vi "Create Controller Names.vi"(0 "Controller name":string, 11 "error in (no error)":errorcluster) -> (4 "Controller Names":string[](array[string]), 15 "error out":errorcluster)   [LabVIEW 2020]
doc: "Create a controller name array from given controller name.\n\nC-887: \nadd additional names for this controller."
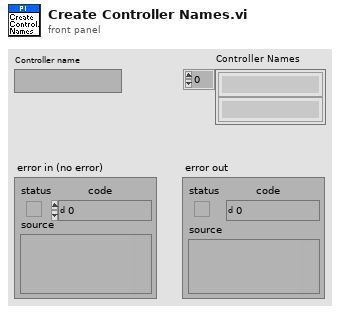
[diagram p1: front panel]
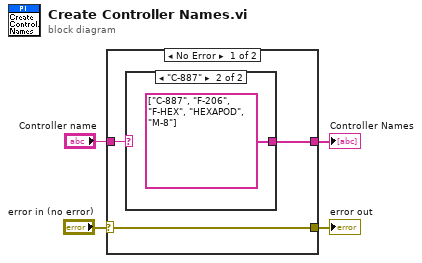
[diagram p0: block diagram]
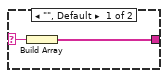
[diagram p2: hidden frame]
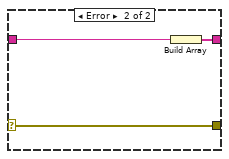
[diagram p3: hidden frame]
diagram:
  n1 = case shown="No Error" "error in (no error)" {
    selector: "error in (no error)" -> [w5 w12]
    tunnel: "Controller name" -> [w7 w13]
    tunnel: [w6 w11] -> w3
    tunnel: [w5 w12] -> w1
    frame No Error {
      n2 = case shown="\"C-887\"" w7 {
        selector: w7 -> [w9 _]
        tunnel: [w8 string[] ["C-887", "F-206", "F-HEX", "HEXAPOD", "M-8"]] -> w6
        frame "", Default {
          n3 = Build Array(w9) -> (w8:string[])
        }
        frame "C-887" {
        }
      }
    }
    frame Error {
      n4 = Build Array(w13) -> (w11:string[])
    }
  }
  "Controller Names" <- w3
  "error out" <- w1
